vi "Set Integer Definition.vi"(10 "Integer Definition":T1, 11 "Integer in":refnum<class "Integer.lvclass">) -> (3 "Integer out":refnum<class "Integer.lvclass">)   [LabVIEW 2020, in "Conditu2.lvlib" / "Columns.lvlib" / "Integer.lvclass"]
uses:
  Integer.lvclass
  Definition.ctl
  Integer.lvclass/Integer.ctl
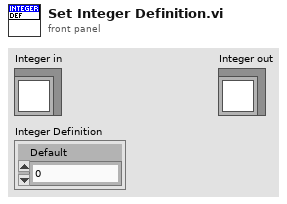
[diagram p1: front panel]
types:
  T1 = typedef "Conditu2.lvlib/Columns.lvlib/Integer.lvclass/Definition.ctl" = cluster{"Default":i64}
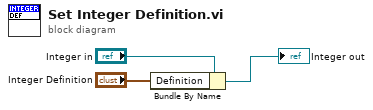
[diagram p0: block diagram]
diagram:
  n1 = Bundle By Name(cluster="Integer in", "Definition"="Integer Definition") -> (→"Integer out":refnum<class "Integer.lvclass">)
